vi "GetSDLCallRefs.vi"(8 "error in (no error)":errorcluster, 11 "VI Refnum":refnum<vi>) -> (0 "error out":errorcluster, 2 "VI SDL Call Nodes":refnum<vi>[](array[refnum]))   [LabVIEW 2024, in "Scripts.lvlib"]
uses:
  Scripts.lvlib
  <vilib>/Utility/error.llb/Clear Errors.vi
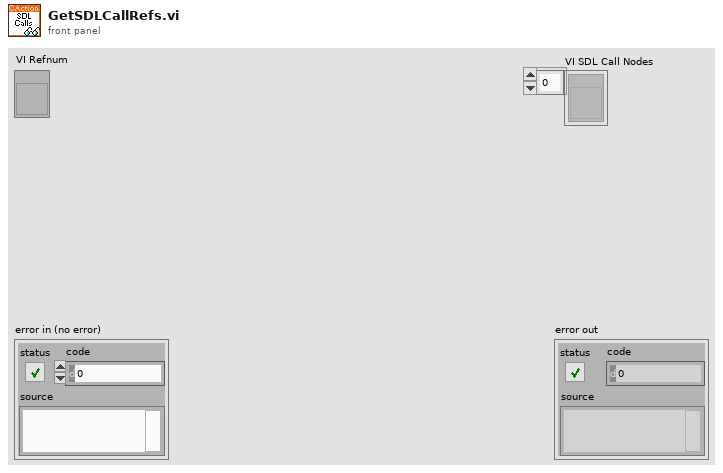
[diagram p1: front panel]
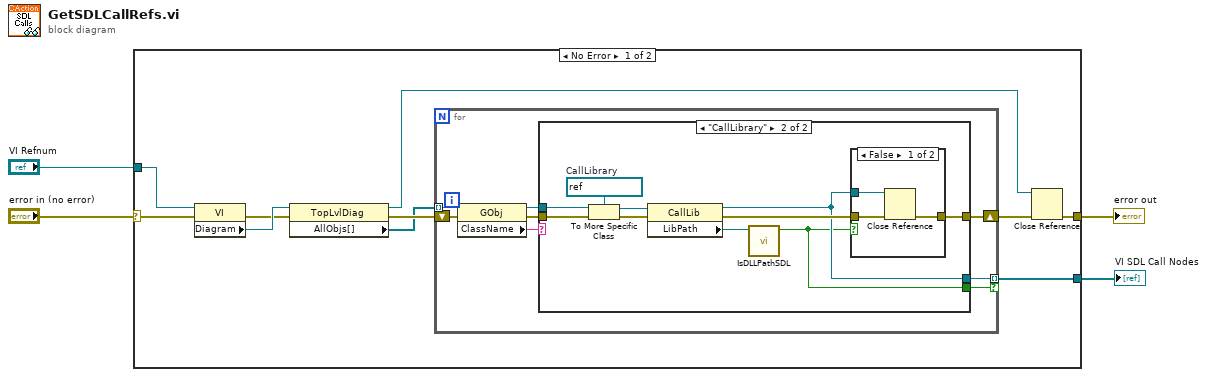
[diagram p0: block diagram]
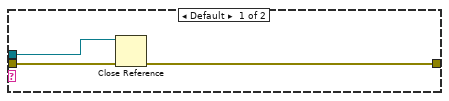
[diagram p2: hidden frame]
diagram:
  n1 = case shown="No Error" "error in (no error)" {
    selector: "error in (no error)" -> [w7 w40]
    tunnel: "VI Refnum" -> [w14 _]
    tunnel: [w6 w40] -> w2
    tunnel: [w5 _] -> w1
    frame No Error {
      n2 = property class="VI"(reference=w14, error in=w7) -> (error out=w12:errorcluster, "Diagram"=w13:refnum<vi>)  [unwired: 1 out]
      n3 = property class="TopLvlDiag"(reference=w13, error in=w12) -> (reference out=w11:refnum<vi>, error out=w10:errorcluster, "AllObjs[]"=w9:refnum<vi>[])
      n4 = for {
        tunnel: w9 -> [w21] mode=indexing
        shift-right: [w19] -> w8
        shift-left: w10 -> [w22]
        tunnel: [w15] -> w5 mode=indexing if=w16
        n5 = property class="GObj"(reference=w21, error in=w22) -> (reference out=w18:refnum<vi>, error out=w20:errorcluster, "ClassName"=w17:string)
        n6 = case shown="\"CallLibrary\"" w17 {
          tunnel: w20 -> [w25 w35]
          tunnel: [w24 w28] -> w19
          tunnel: w18 -> [w23 w34]
          tunnel: [_ w26] -> w16
          tunnel: [_ w27] -> w15
          frame Default {
            n7 = Close Reference(reference=w23, error in (no error)=w25) -> (error out=w24:errorcluster)
          }
          frame "CallLibrary" {
            w33 = refnum<vi> refnum  # CallLibrary
            n8 = To More Specific Class(target class=w33, reference=w34, error in=w35) -> (specific class reference=w31:refnum<vi>, error out=w32:errorcluster)
            n9 = property class="CallLib"(reference=w31, error in=w32) -> (reference out=w27:refnum<vi>, error out=w30:errorcluster, "LibPath"=w29:path)
            n10 = call "IsDLLPathSDL.vi"("DLL Path"=w29) -> ("Is SDL?"=w26:bool)  [unwired: 8 in, 2 out]
            n11 = case shown="False" w26 {
              tunnel: w30 -> [w38 w39]
              tunnel: [w37 w39] -> w28
              tunnel: w27 -> [w36 _]
              frame False {
                n12 = Close Reference(reference=w36, error in (no error)=w38) -> (error out=w37:errorcluster)
              }
              frame True {
              }
            }
          }
        }
      }
      n13 = Close Reference(reference=w11, error in (no error)=w8) -> (error out=w6:errorcluster)
    }
    frame Error {
    }
  }
  "error out" <- w2
  "VI SDL Call Nodes" <- w1
